vi "StepConvertToMES Step.vi"(10 "Step":string) -> (2 "MES Step":string)   [LabVIEW 2012]
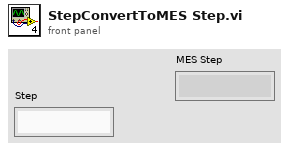
[diagram p1: front panel]
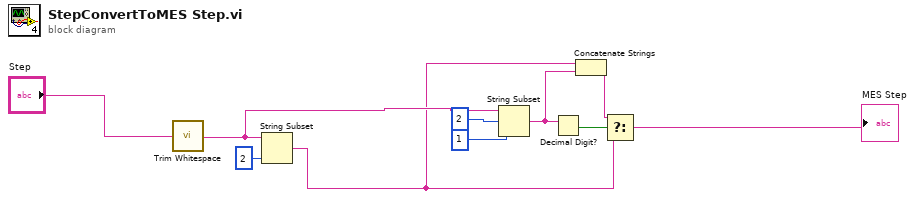
[diagram p0: block diagram]
diagram:
  n1 = call <vilib>:"Trim Whitespace.vi"("string"="Step") -> ("trimmed string"=w9:string)  [unwired: 1 in]
  n2 = String Subset(string=w9, length (rest)=2 ("length (rest)")) -> (substring=w3:string)  [unwired: 1 in]
  n3 = String Subset(string=w9, offset (0)=2, length (rest)=1 ("length (rest)")) -> (substring=w5:string)
  n4 = Decimal Digit?(1:w5) -> (0:w6:bool)
  n5 = Concatenate Strings(w3, w5) -> (w4:string)
  n6 = Select(t=w4, s=w6, f=w3) -> (s? t:f=→"MES Step":string)
